vi "TCP_write.vi"(8 "error in":errorcluster, 9 "Parameter 2":string, 10 "Parameter 1":string="FL", 11 "connection ID":refnum<k5>) -> (0 "error out":errorcluster, 2 "Driver response":bool, 3 "TCP Network Connection out":refnum<k5>)   [LabVIEW 2019]
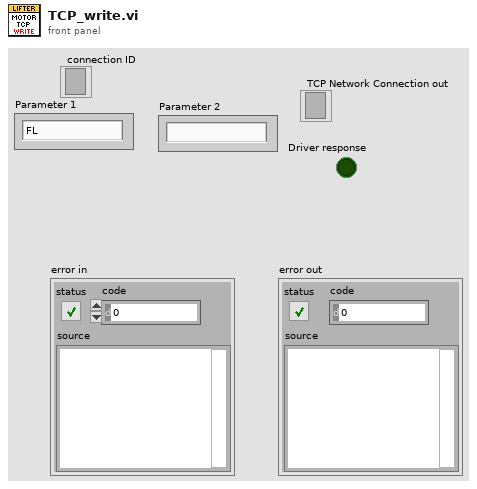
[diagram p1: front panel]
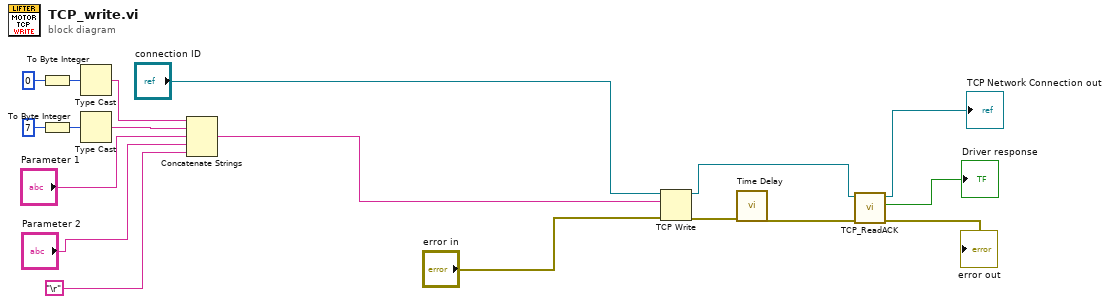
[diagram p0: block diagram]
diagram:
  n1 = To Byte Integer(number=i8 0) -> (8bit integer=w15:i8)
  n2 = To Byte Integer(number=i8 7) -> (8bit integer=w18:i8)
  n3 = Type Cast(x=w15) -> (*(type *) &x=w16:string)  [unwired: 1 in]
  n4 = Type Cast(x=w18) -> (*(type *) &x=w17:string)  [unwired: 1 in]
  n5 = Concatenate Strings(w16, w17, "Parameter 1", "Parameter 2", "\r") -> (w1:string)
  n6 = TCP Write(connection ID="connection ID", data in=w1, error in (no error)="error in") -> (connection ID out=w5:refnum<k5>, error out=w9:errorcluster)  [unwired: 1 in, 1 out]
  n7 = call "Time Delay"("error in (no error)"=w9) -> ("error out"=w8:errorcluster)  [unwired: 10 in]
  n8 = call "TCP_ReadACK.vi"("error in (no error)"=w8, "TCP Network Connection in"=w5) -> ("error out"=→"error out":errorcluster, "Driver response"=→"Driver response":bool, "TCP Network Connection out"=→"TCP Network Connection out":refnum<k5>)  [unwired: 7 in]
